vi "CalculatorVIMarcoGonzalez.vi"() -> ()   [LabVIEW 2012]
doc: "This VI can take the square root of a number, square the number, add 2 numbers, subtract 2 numbers, multiply 2 numbers, divide 2 numbers, raise a number to a power, reciprocal of a number."
panel:
  in  "?":bool
  in  "?":u16(ring) items=["Square Root", "Square", "Addition", "Substraction", "Multiplication", "Division", "Raise to the Power", "Reciprocal"]
  out "Z":dbl
  in  "Y":dbl
  in  "X":dbl
  # "Marco Gonzalez\nEA3\n02/09/2017"
  # "="
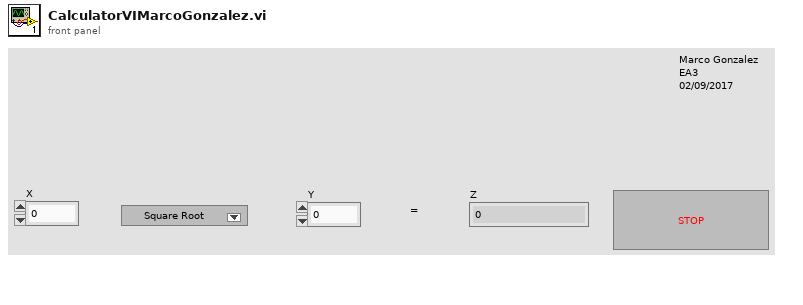
[diagram p1: front panel]
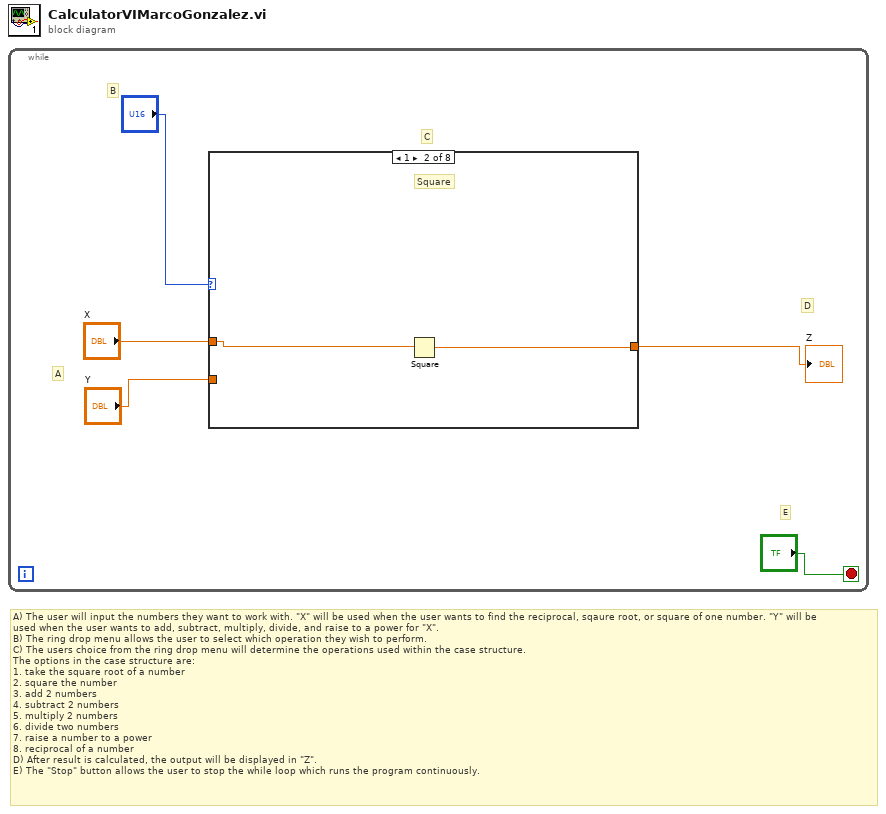
[diagram p0: block diagram]
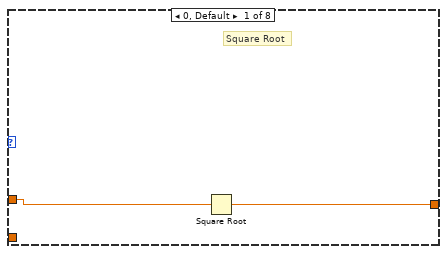
[diagram p2: hidden frame]
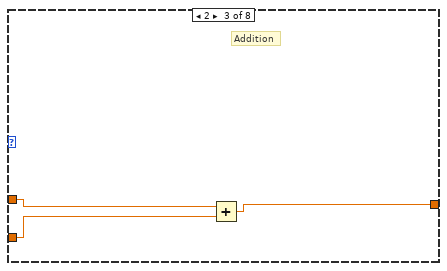
[diagram p3: hidden frame]
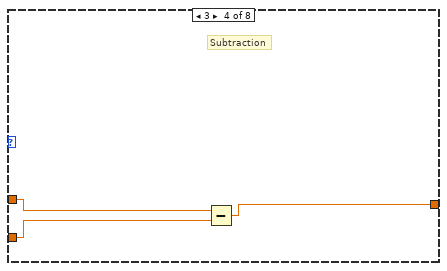
[diagram p4: hidden frame]
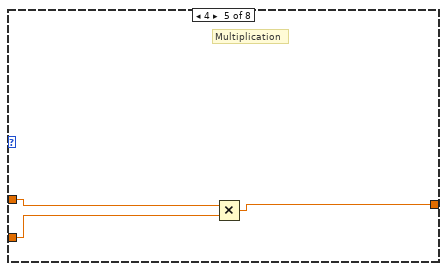
[diagram p5: hidden frame]
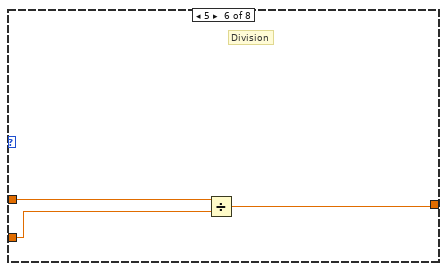
[diagram p6: hidden frame]
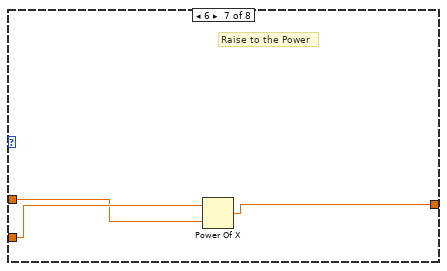
[diagram p7: hidden frame]
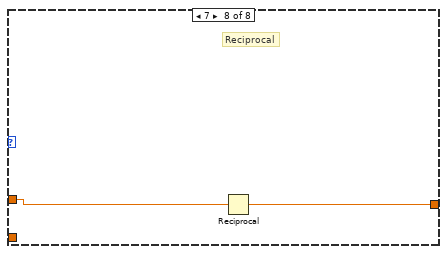
[diagram p8: hidden frame]
diagram:
  # "A) The user will input the numbers they want to work with. \"X\" will be used when the user wants to find the reciprocal, sqaure root, or square of one number. \"Y\" will be\nused when the user wants to add, subtract, multiply, divide, and raise to a power for \"X\".\nB) The ring drop menu allows the user to select which operation they wish to perform. \nC) The users choice from the ring drop menu will determine the operations used within the case structure.\nThe options in the case structure are: \n1. take the square root of a number\n2. square the number\n3. add 2 numbers\n4. subtract 2 numbers\n5. multiply 2 numbers\n6. divide two numbers\n7. raise a number to a power\n8. reciprocal of a number\nD) After result is calculated, the output will be displayed in \"Z\".\nE) The \"Stop\" button allows the user to stop the while loop which runs the program continuously."
  n1 = while {
    stop <- "?" stop-if-true
    # "E"
    # "D"
    # "C"
    # "B"
    # "A"
    n2 = case shown="1" "?" {
      tunnel: "X" -> [w7 w9 w11 w14 w18 w20 w23 w26]
      tunnel: [w6 w8 w10 w13 w16 w19 w22 w25] -> w4
      tunnel: "Y" -> [_ _ w12 w15 w17 w21 w24 _]
      frame 0, Default {
        # "Square Root"
        n3 = Square Root(x=w7) -> (sqrt(x)=w6:dbl)
      }
      frame 1 {
        # "Square"
        n4 = Square(x=w9) -> (x^2=w8:dbl)
      }
      frame 2 {
        # "Addition"
        n5 = Add(x=w11, y=w12) -> (x+y=w10:dbl)
      }
      frame 3 {
        # "Subtraction"
        n6 = Subtract(x=w14, y=w15) -> (x-y=w13:dbl)
      }
      frame 4 {
        # "Multiplication"
        n7 = Multiply(x=w18, y=w17) -> (x*y=w16:dbl)
      }
      frame 5 {
        # "Division"
        n8 = Divide(x=w20, y=w21) -> (x/y=w19:dbl)
      }
      frame 6 {
        # "Raise to the Power"
        n9 = Power Of X(1:w23, 2:w24) -> (0:w22:dbl)
      }
      frame 7 {
        # "Reciprocal"
        n10 = Reciprocal(x=w26) -> (1/x=w25:dbl)
      }
    }
    "Z" <- w4
  }
